vi "Fit.vi"(8 "error in (no error)":errorcluster caption="entrée d'erreur (pas d'erreur)", 9 "y":string[][](array[string]), 10 "X":string[][](array[string]), 11 "Binarizer en entrée":refnum<class "Binarizer.lvclass">) -> (0 "error out":errorcluster caption="sortie d'erreur", 2 "String Data":string, 3 "Binarizer en sortie":refnum<class "Binarizer.lvclass">)   [LabVIEW 2020, in "Binarizer.lvclass"]
doc: "This method is just there to implement the usual API and hence work in pipelines.\n\nReturns : \n\n- String : OK"
uses:
  Binarizer.lvclass
  Binarizer.lvclass/Binarizer.ctl
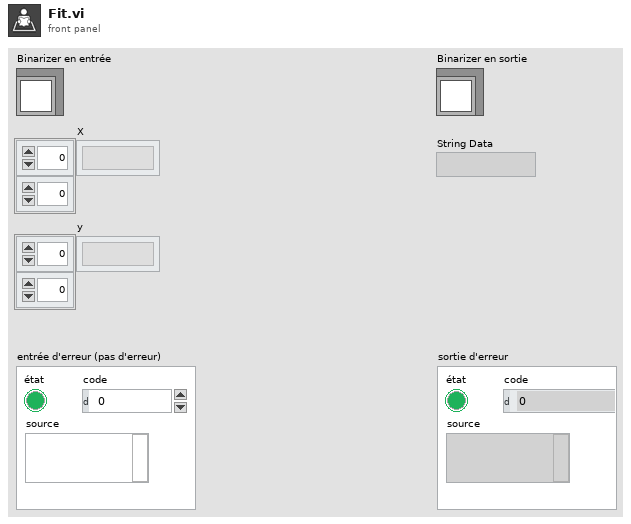
[diagram p1: front panel]
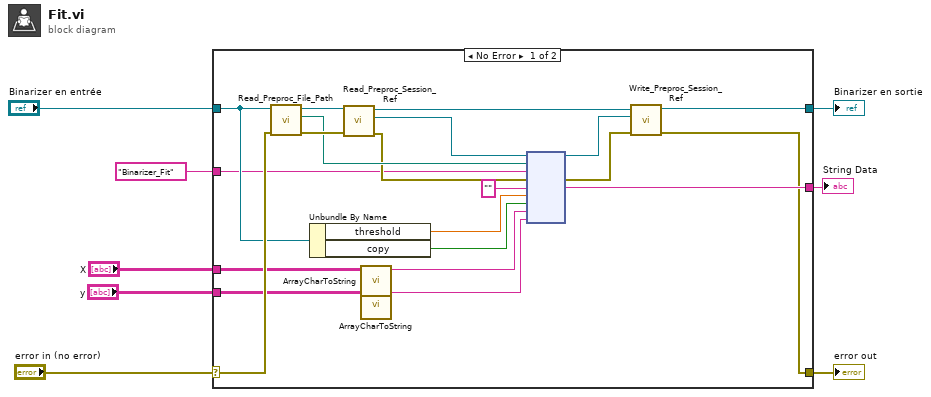
[diagram p0: block diagram]
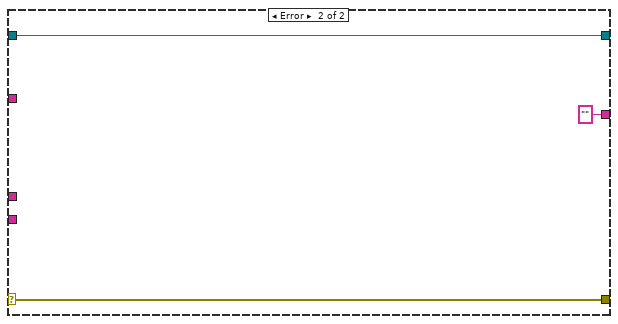
[diagram p2: hidden frame]
diagram:
  n1 = case shown="No Error" "error in (no error)" {
    selector: "error in (no error)" -> [w18 w32]
    tunnel: [w10 w32] -> w7
    tunnel: [w9 w31] -> w5
    tunnel: "Binarizer en entrée" -> [w17 w31]
    tunnel: "X" -> [w14 _]
    tunnel: "y" -> [w13 _]
    tunnel: "Binarizer_Fit" -> [w16 _]
    tunnel: [w15 ""] -> w1
    frame No Error {
      n2 = call-dynamic "Read_Preproc_File_Path.vi"("error in (no error)"=w18, "Python in"=w17) -> ("error out"=w28:errorcluster, "File_Path"=w25:path, "Python out"=w29:refnum<class "Binarizer.lvclass">)  [unwired: 7 in]
      n3 = Unbundle By Name(w17) -> ("threshold"=w20:dbl, "copy"=w19:bool)
      n4 = call-dynamic "Read_Preproc_Session_Ref.vi"("error in (no error)"=w28, "Python in"=w29) -> ("error out"=w24:errorcluster, "Session_ref"=w26:refnum<k35>, "Python out"=w27:refnum<class "Binarizer.lvclass">)  [unwired: 7 in]
      n5 = call "ArrayCharToString.vi"("TAB"=w14) -> ("Instruction"=w12:string)  [unwired: 10 in]
      n6 = call "ArrayCharToString.vi"("TAB"=w13) -> ("Instruction"=w11:string)  [unwired: 10 in]
      n7 = node(w26, w25, w16, w24, "", w20, w19, w12, w11) -> (w22:refnum<k35>, w23:errorcluster, w15:string)  [unwired: 4 in, 2 out]
      n8 = call-dynamic "Write_Preproc_Session_Ref.vi"("error in (no error)"=w23, "Session_ref"=w22, "Python in"=w27) -> ("error out"=w10:errorcluster, "Python out"=w9:refnum<class "Binarizer.lvclass">)  [unwired: 7 in]
    }
    frame Error {
    }
  }
  "error out" <- w7
  "Binarizer en sortie" <- w5
  "String Data" <- w1
